vi "Check Device Support.vi"(7 "Output Error?":bool, 8 "error in (no error)":errorcluster, 11 "Potentiostat Galvanostat in":refnum<class "Potentiostat Galvanostat.lvclass">) -> (0 "error out":errorcluster, 1 "Is supported?":bool, 3 "Potentiostat Galvanostat out":refnum<class "Potentiostat Galvanostat.lvclass">)   [LabVIEW 2018, in "Potentiostat Galvanostat.lvclass"]
uses:
  Potentiostat Galvanostat.lvclass
  Potentiostat Galvanostat.lvclass/Potentiostat Galvanostat.ctl
  Controls/Error Codes.ctl
  BL_GetErrorMsg.vi
  <vilib>/Utility/error.llb/Error Cluster From Error Code.vi
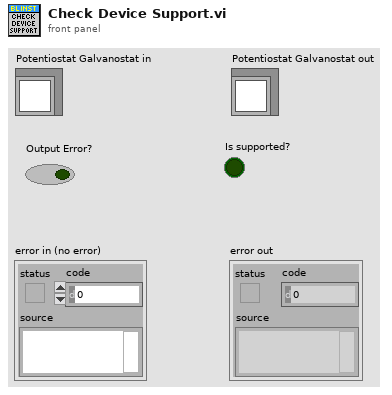
[diagram p1: front panel]
types:
  T1 = typedef "Potentiostat Galvanostat.lvclass/Error Codes.ctl" = i32
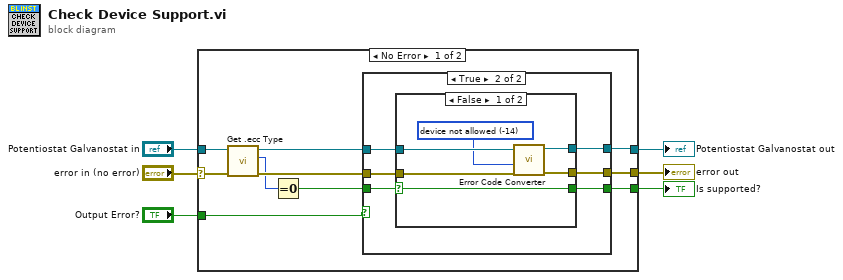
[diagram p0: block diagram]
diagram:
  n1 = case shown="No Error" "error in (no error)" {
    selector: "error in (no error)" -> [w15 w36]
    tunnel: [w10 w36] -> w5
    tunnel: [w11 w35] -> w3
    tunnel: "Potentiostat Galvanostat in" -> [w16 w35]
    tunnel: "Output Error?" -> [w8 _]
    tunnel: [w9 _] -> w1
    frame No Error {
      n2 = call "Get .ecc Type.vi"("error in (no error)"=w15, "Potentiostat Galvanostat in"=w16) -> ("error out"=w13:errorcluster, "Ecc Type"=w7:enum16{"ecc", "ecc4"}, "Potentiostat Galvanostat out"=w14:refnum<class "Potentiostat Galvanostat.lvclass">)  [unwired: 6 in, 1 out]
      n3 = Equal To 0?(x=w7) -> (x = 0?=w12:bool)
      n4 = case shown="True" w8 {
        tunnel: w14 -> [w17 w25]
        tunnel: w13 -> [w18 w24]
        tunnel: w12 -> [w19 w21]
        tunnel: [w19 w20] -> w9
        tunnel: [w17 w23] -> w11
        tunnel: [w18 w22] -> w10
        frame False {
        }
        frame True {
          n5 = case shown="False" w21 {
            selector: w21 -> [w26 w32]
            tunnel: w25 -> [w31 w34]
            tunnel: w24 -> [w29 w33]
            tunnel: [w28 w34] -> w23
            tunnel: [w27 w33] -> w22
            tunnel: [w26 w32] -> w20
            frame False {
              w30 = T1 -14 items=["No Error"=0, "no instrument connected"=-1, "connection in progress"=-2, "selected channel(s) unplugged"=-3, "invalid function parameters"=-4, "selected file does not exist"=-5, "function failed"=-6, "no channel selected"=-7, "invalid instrument configuration"=-8, "EC-Lab firmware loaded on the instrument"=-9, "library not correctly loaded in memory"=-10, "USB library not correctly loaded in memory"=-11, "function of the library already in progress"=-12, "selected channel(s) already used"=-13, "device not allowed"=-14, "Invalid update function parameters"=-15, "internal instrument communication failed"=-101, "too many data to transfer from the instrument (device error)"=-102, "selected channel(s) unplugged (device error)"=-103, "instrument response error"=-104, "invalid message size"=-105] ("Error Code")
              n6 = call "Error Code Converter.vi"("error in (no error)"=w29, "Error Code"=w30, "Potentiostat Galvanostat in"=w31) -> ("error out"=w27:errorcluster, "Potentiostat Galvanostat out"=w28:refnum<class "Potentiostat Galvanostat.lvclass">)  [unwired: 7 in]
            }
            frame True {
            }
          }
        }
      }
    }
    frame Error {
    }
  }
  "error out" <- w5
  "Potentiostat Galvanostat out" <- w3
  "Is supported?" <- w1
